vi "Define Label.vi"(4 "error in (no error)":errorcluster, 6 "Number of Label":i32=1 min=1 max=100, 7 "VISA resource name":refnum<visa-resource-name>) -> (0 "error out":errorcluster, 3 "VISA resource name out":refnum<visa-resource-name>)   [LabVIEW 2014, in "Newport ESP301.lvlib"]
doc: "This command defines a label inside a program. In combination with JL (jump to label) command, they offer significant program flow control.\nThe operation of the DL / JL command pair is similar to commands in other\ncomputer languages that allow conditional jumps (or GOTO's) to predefined labels in a program.\nNote:\nThis command does not generate an error when not used inside a program. Since it can not do any harm, it is only ignored."
uses:
  Newport ESP301.lvlib
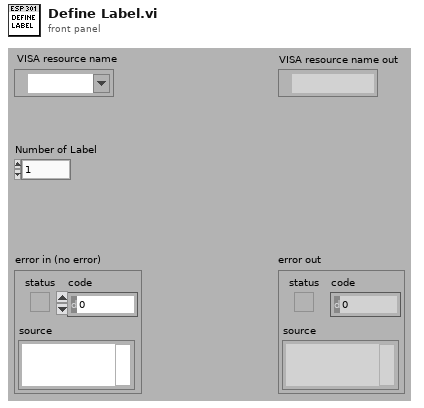
[diagram p1: front panel]
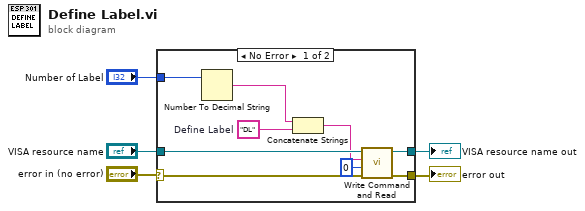
[diagram p0: block diagram]
diagram:
  n1 = case shown="No Error" "error in (no error)" {
    selector: "error in (no error)" -> [w11 w16]
    tunnel: [w13 w16] -> w5
    tunnel: "VISA resource name" -> [w14 w15]
    tunnel: [w12 w15] -> w4
    tunnel: "Number of Label" -> [w10 _]
    frame No Error {
      w9 = "DL"  # Define Label
      n2 = Number To Decimal String(number=w10) -> (decimal integer string=w8:string)  [unwired: 1 in]
      n3 = Concatenate Strings(w8, w9) -> (w7:string)
      n4 = call "Write Command and Read.vi"("error in (no error)"=w11, "Bytes to read (100)"=u32 0, "Command"=w7, "VISA resource name"=w14) -> ("error out"=w13:errorcluster, "VISA resource name out"=w12:refnum<visa-resource-name>)  [unwired: 3 in, 1 out]
    }
    frame Error {
    }
  }
  "error out" <- w5
  "VISA resource name out" <- w4
